vi "Read Commands.vi"(8 "error in (no error)":errorcluster, 11 "Iteration Actions in":refnum<class "Iteration Actions.lvclass">) -> (0 "error out":errorcluster, 1 "Analog Commands":map{refnum<class "MessageQ.lvclass">, T1[]}(c390), 2 "Digital Commands":map{refnum<class "MessageQ.lvclass">, T2[]}(c390), 3 "Iteration Actions out":refnum<class "Iteration Actions.lvclass">)   [LabVIEW 2020, in "VolatusSeq.lvlib" / "Iteration Actions.lvclass"]
uses:
  Iteration Actions.lvclass
  Iteration Actions.lvclass/Iteration Actions.ctl
  Volatus/MessageQ/MessageQ.lvclass
  messages/CmdDigital/Data.ctl
  messages/CmdDigital/CmdDigital.lvlib
  messages/CmdAnalog/Data.ctl
  messages/CmdAnalog/CmdAnalog.lvlib
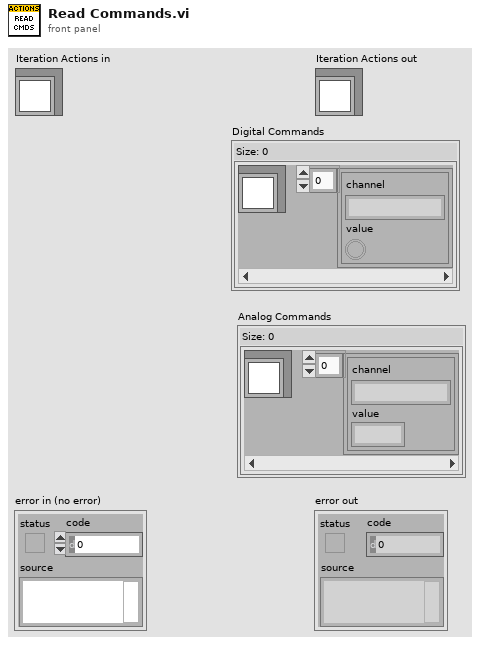
[diagram p1: front panel]
types:
  T1 = typedef "CmdAnalog.lvlib/Data.ctl" = cluster{"channel":string, "value":dbl}
  T2 = typedef "CmdDigital.lvlib/Data.ctl" = cluster{"channel":string, "value":bool}
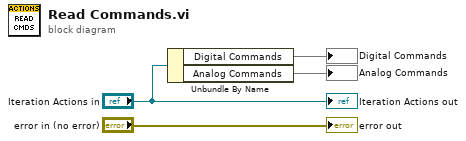
[diagram p0: block diagram]
diagram:
  n1 = Unbundle By Name("Iteration Actions in") -> ("Digital Commands"=→"Digital Commands":map{refnum<class "MessageQ.lvclass">, T2[]}, "Analog Commands"=→"Analog Commands":map{refnum<class "MessageQ.lvclass">, T1[]})
  "error out" <- "error in (no error)"
  "Iteration Actions out" <- "Iteration Actions in"
